vi "cam0-角度换算0到360.vi"() -> ()   [LabVIEW 2015]
panel:
  out "角度输出":sgl
  in  "角度输入":sgl
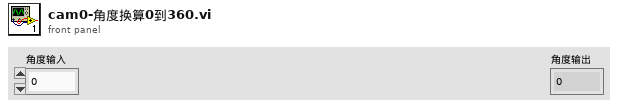
[diagram p1: front panel]
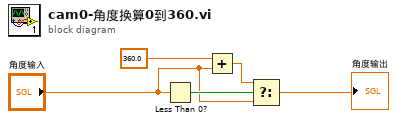
[diagram p0: block diagram]
diagram:
  n1 = Less Than 0?(x="角度输入") -> (x < 0?=w5:bool)
  n2 = Add(x=sgl 360.0, y="角度输入") -> (x+y=w3:sgl)
  n3 = Select(t=w3, s=w5, f="角度输入") -> (s? t:f=→"角度输出":sgl)
